vi "DB_Select.vi"() -> ()   [LabVIEW 2020]
uses:
  <vilib>/addons/database/Connection.llb/DB Tools Open Connec (String).vi
  <vilib>/addons/database/NI_Database_API.lvlib
panel:
  out "Table_ID":string[][](array[string])
  out "data":variant[][](array[variant])
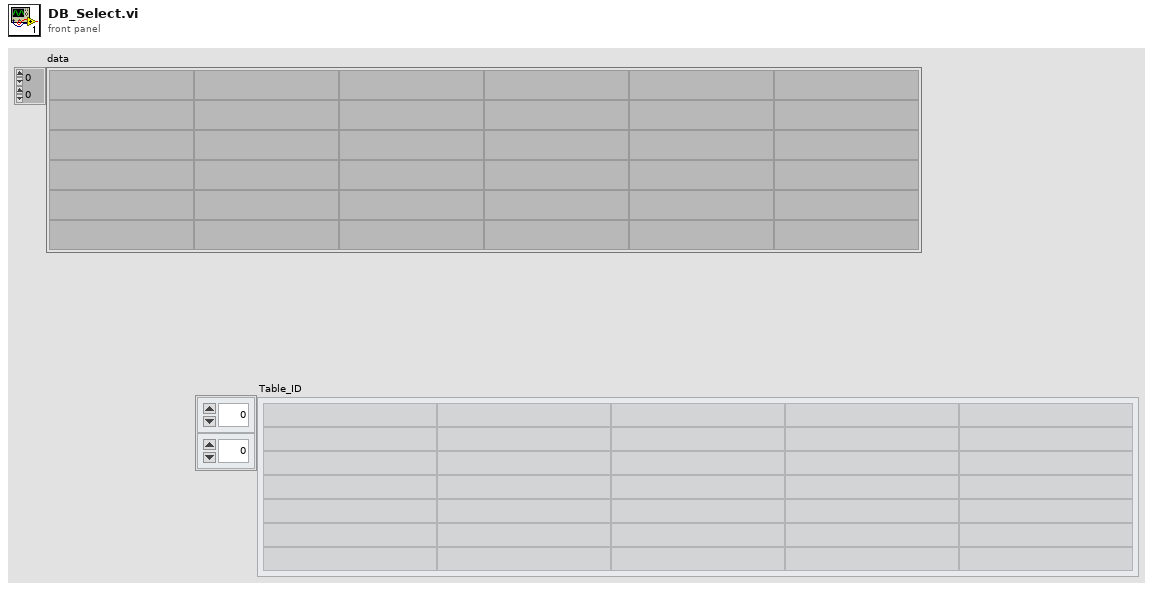
[diagram p1: front panel]
types:
  T1 = typedef "NI_Database_API.lvlib/Conn ObjectReference.ctl" = refnum<k1>
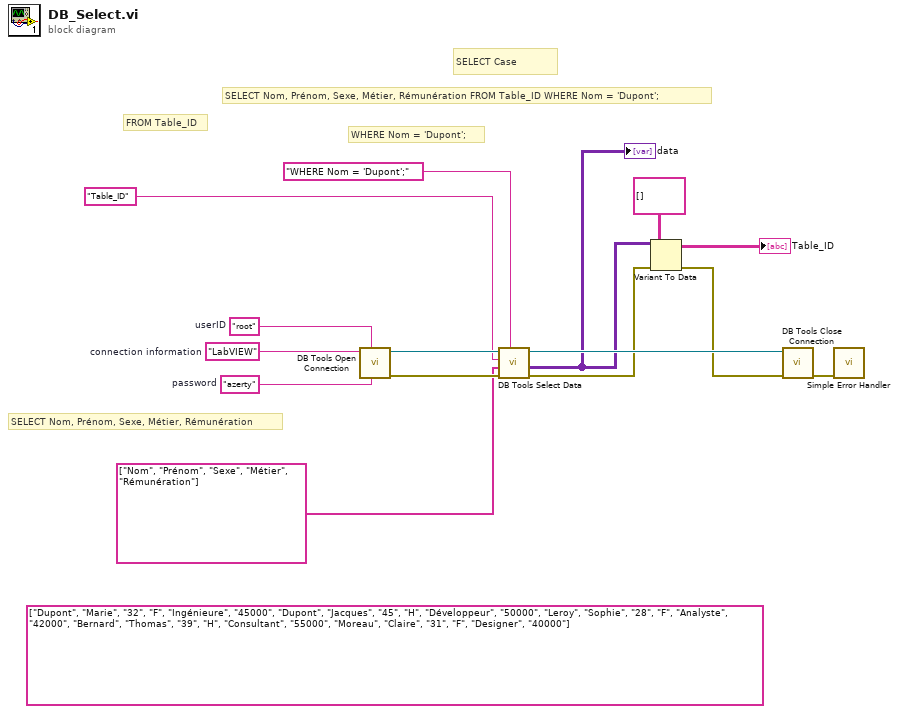
[diagram p0: block diagram]
diagram:
  w1 = "azerty"  # password
  w2 = "root"  # userID
  (unwired) string[][] [["Dupont", "Marie", "32", "F", "Ingénieure", "45000"], ["Dupont", "Jacques", "45", "H", "Développeur", "50000"], ["Leroy", "Sophie", "28", "F", "Analyste", "42000"], ["Bernard", "Thomas", "39", "H", "Consultant", "55000"], ["Moreau", "Claire", "31", "F", "Designer", "40000"]] ("data 2")
  w3 = "LabVIEW"  # connection information
  # "WHERE Nom = 'Dupont';"
  # "FROM Table_ID"
  # "SELECT Nom, Prénom, Sexe, Métier, Rémunération"
  # "SELECT Nom, Prénom, Sexe, Métier, Rémunération FROM Table_ID WHERE Nom = 'Dupont';"
  # "SELECT Case"
  n1 = call-poly <vilib>:"DB Tools Open Connection.vi"("password"=w1, "userID"=w2, "connection information"=w3) -> ("error out"=w14:errorcluster, "connection reference"=w13:T1)  [unwired: 5 in]
  n2 = call <vilib>:"DB Tools Select Data.vi"("condition"="WHERE Nom = 'Dupont';", "error in (no error)"=w14, "columns"=string[] ["Nom", "Prénom", "Sexe", "Métier", "Rémunération"], "table"="Table_ID", "connection reference"=w13) -> ("error out"=w8:errorcluster, "data"=w9:variant[][], "connection reference out"=w11:T1)  [unwired: 1 in]
  "data" <- w9
  n3 = Variant To Data(error in=w8, type=string[][] [], Variant=w9) -> (data=→"Table_ID":string[][], error out=w7:errorcluster)
  n4 = call <vilib>:"DB Tools Close Connection.vi"("error in (no error)"=w7, "connection reference"=w11) -> ("error out"=w15:errorcluster)  [unwired: 5 in]
  n5 = call <vilib>:"Simple Error Handler.vi"("error in (no error)"=w15) -> ()  [unwired: 4 in, 5 out]
